vi "Read Cleanliness.vi"(8 "error in (no error)":errorcluster, 11 "Nigel Tamagotchi in":refnum<class "Tamagotchi Full Actor.lvclass">) -> (0 "error out":errorcluster, 2 "Cleanliness":i16=100, 3 "Nigel Tamagotchi out":refnum<class "Tamagotchi Full Actor.lvclass">)   [LabVIEW 2026, in "Tamagotchi Full Actor.lvclass"]
uses:
  Tamagotchi Full Actor.lvclass
  Tamagotchi Full Actor.lvclass/Tamagotchi Full Actor.ctl
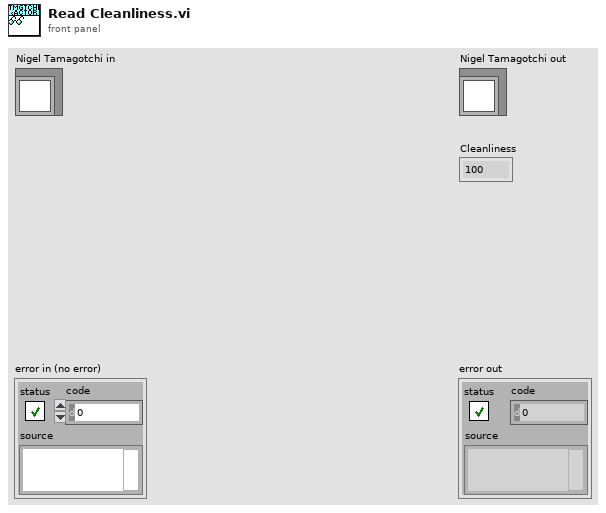
[diagram p1: front panel]
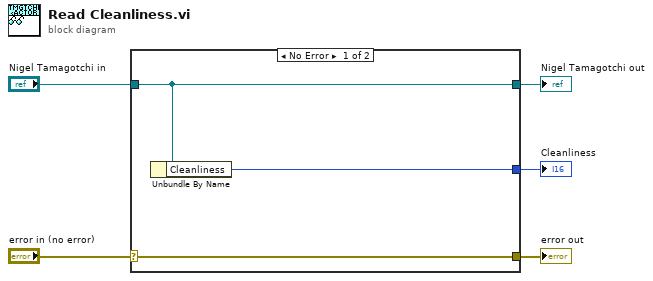
[diagram p0: block diagram]
diagram:
  n1 = case shown="No Error" "error in (no error)" {
    selector: "error in (no error)" -> [w8 w9]
    tunnel: [w8 w9] -> w4
    tunnel: [w7 w10] -> w2
    tunnel: "Nigel Tamagotchi in" -> [w7 w10]
    tunnel: [w6 _] -> w1
    frame No Error {
      n2 = Unbundle By Name(w7) -> ("Cleanliness"=w6:i16)
    }
    frame Error {
    }
  }
  "error out" <- w4
  "Nigel Tamagotchi out" <- w2
  "Cleanliness" <- w1
